vi "LiftEncoders.vi"(1 "Terms":i32) -> ()   [LabVIEW 2017]
uses:
  Robot Global Data.vi
panel:
  out "Position":dbl(graph)
  out "Velocity":dbl(graph)
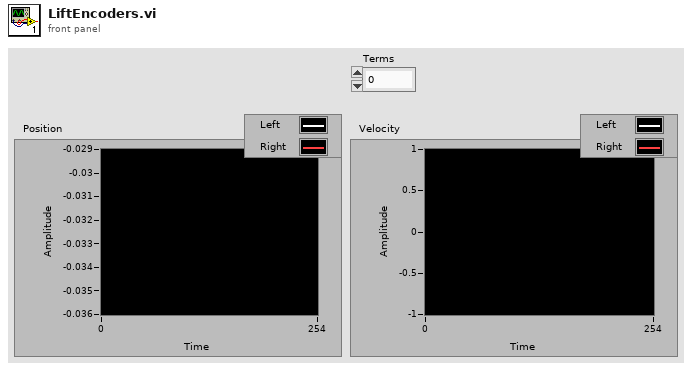
[diagram p1: front panel]
types:
  T1 = typedef "WPI_EncoderDevRef.ctl" = cluster{"DevStatus":errorcluster, "EncoderIndex":T2, "CounterIndex":T3, "DistancePerCount":dbl, "Decoding Type":T4}
  T2 = typedef "FPGA_EncoderIdx.ctl" = enum8{"Enc 0", "Enc 1", "Enc 2", "Enc 3", "Enc 4", "Enc 5", "Enc 6", "Enc 7", "Invalid"}
  T3 = typedef "FPGA_CounterCtrSystemIndex.ctl" = enum8{"Ctr 0", "Ctr 1", "Ctr 2", "Ctr 3", "Ctr 4", "Ctr 5", "Ctr 6", "Ctr 7", "Invalid"}
  T4 = typedef "WPI_EncoderType.ctl" = enum16{"1x", "2x", "4x"}
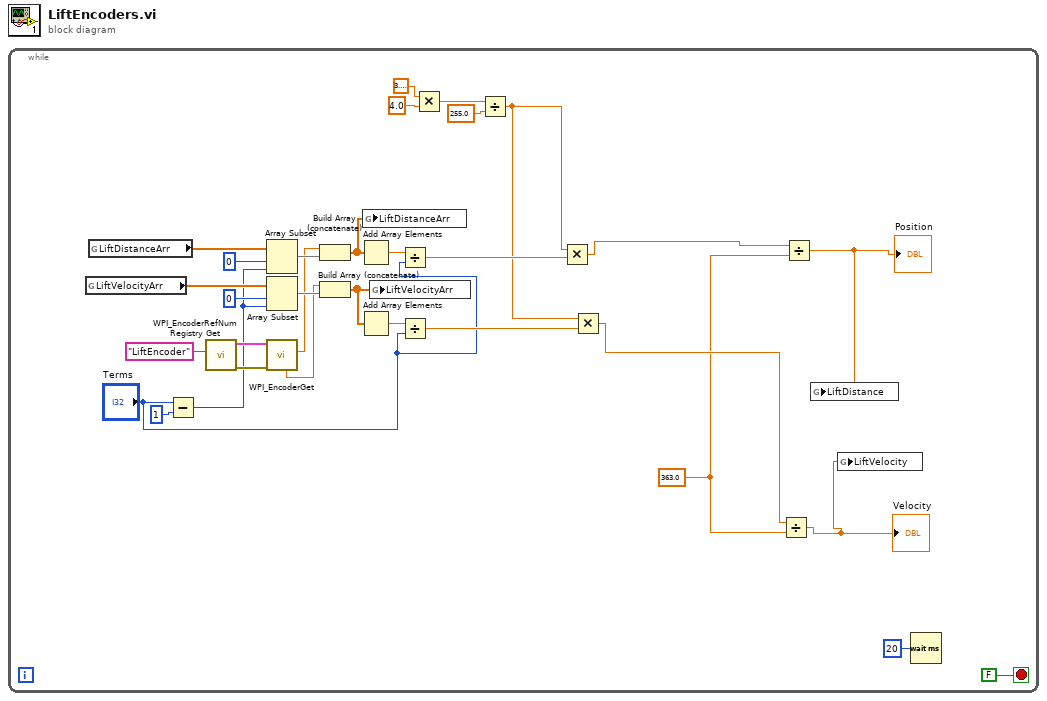
[diagram p0: block diagram]
diagram:
  n1 = while {
    stop <- FALSE stop-if-true
    w6 = 363.0
    n2 = global read "Robot Global Data.vi" "LiftVelocityArr"() -> (w27:dbl[])
    n3 = global read "Robot Global Data.vi" "LiftDistanceArr"() -> (w29:dbl[])
    n4 = Subtract(x="Terms", y=1) -> (x-y=w23:i32)
    n5 = call <vilib>:"WPI_EncoderRefNum Registry Get.vi"("refnum name"="LiftEncoder") -> ("error out"=w31:errorcluster, "EncoderDevRef"=w32:T1)  [unwired: 9 in]
    n6 = Array Subset(array=w29, index=0, length=w23) -> (w25:dbl[])
    n7 = Array Subset(array=w27, index=0, length=w23) -> (w22:dbl[])
    n8 = call <vilib>:"WPI_EncoderGet.vi"("error in (no error)"=w31, "EncoderDevRef"=w32) -> ("Distance"=w17:dbl, "Rate"=w16:dbl)  [unwired: 4 in, 4 out]
    n9 = Build Array (concatenate)(w17, w25) -> (w21:dbl[])
    n10 = Build Array (concatenate)(w16, w22) -> (w20:dbl[])
    n11 = Add Array Elements(numeric array=w21) -> (sum=w19:dbl)
    n12 = Add Array Elements(numeric array=w20) -> (sum=w18:dbl)
    n13 = global write "Robot Global Data.vi" "LiftDistanceArr"(w21) -> ()
    n14 = global write "Robot Global Data.vi" "LiftVelocityArr"(w20) -> ()
    n15 = Divide(x=w19, y="Terms") -> (x/y=w11:dbl)
    n16 = Divide(x=w18, y="Terms") -> (x/y=w10:dbl)
    n17 = Multiply(x=3.141592653589793, y=4.0) -> (x*y=w13:dbl)
    n18 = Divide(x=w13, y=255.0) -> (x/y=w9:dbl)
    n19 = Multiply(x=w9, y=w11) -> (x*y=w8:dbl)
    n20 = Multiply(x=w9, y=w10) -> (x*y=w7:dbl)
    n21 = Divide(x=w7, y=w6) -> (x/y=w1:dbl)
    "Velocity" <- w1
    n22 = Divide(x=w8, y=w6) -> (x/y=w2:dbl)
    "Position" <- w2
    n23 = global write "Robot Global Data.vi" "LiftDistance"(w2) -> ()
    n24 = global write "Robot Global Data.vi" "LiftVelocity"(w1) -> ()
    n25 = Wait (ms)(milliseconds to wait=u32 20) -> ()  [unwired: 1 out]
  }
